vi "MESLog_Detail_Result.vi"(0 "DetailResultID":string, 1 "ItemResultID":string, 2 "Barcode":string, 3 "LoopID":string, 4 "BeginDate":string, 5 "DiffTime":string, 6 "EndDate":string, 7 "Description":string, 8 "DetailResult":string, 10 "CreateDate":string) -> (16 "Detail_Result":string)   [LabVIEW 2014]
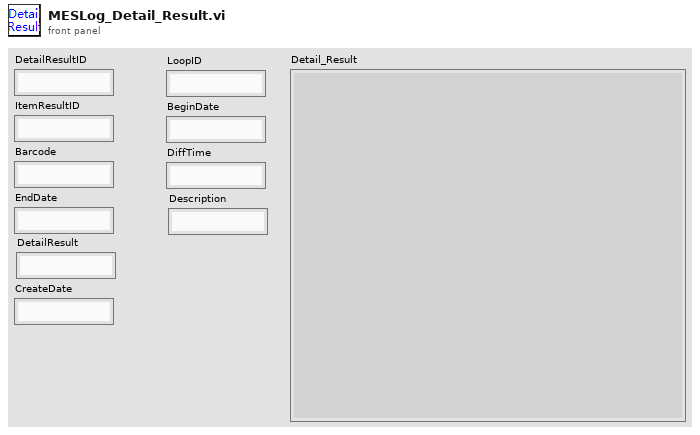
[diagram p1: front panel]
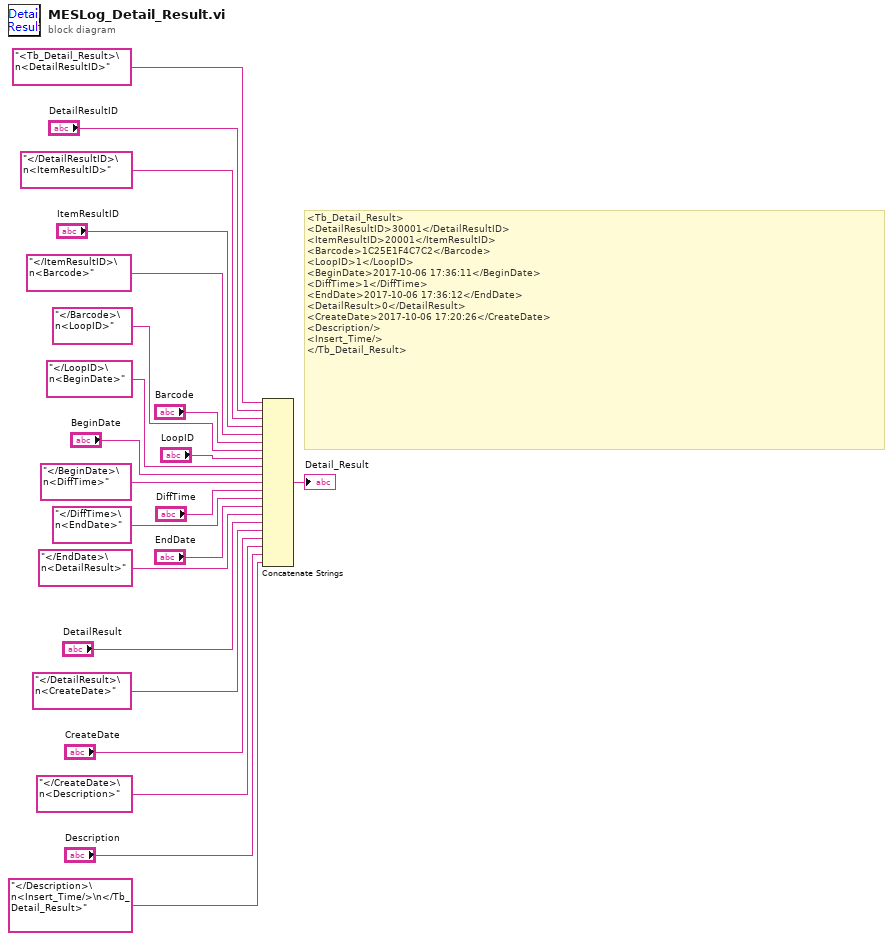
[diagram p0: block diagram]
diagram:
  # "<Tb_Detail_Result>\n<DetailResultID>30001</DetailResultID>\n<ItemResultID>20001</ItemResultID>\n<Barcode>1C25E1F4C7C2</Barcode>\n<LoopID>1</LoopID>\n<BeginDate>2017-10-06 17:36:11</BeginDate>\n<DiffTime>1</DiffTime>\n<EndDate>2017-10-06 17:36:12</EndDate>\n<DetailResult>0</DetailResult>\n<CreateDate>2017-10-06 17:20:26</CreateDate>\n<Description/>\n<Insert_Time/>\n</Tb_Detail_Result>"
  n1 = Concatenate Strings("<Tb_Detail_Result>\n<DetailResultID>" ("string"), "DetailResultID", "</DetailResultID>\n<ItemResultID>" ("string"), "ItemResultID", "</ItemResultID>\n<Barcode>" ("string"), "Barcode", "</Barcode>\n<LoopID>" ("string"), "LoopID", "</LoopID>\n<BeginDate>" ("string"), "BeginDate", "</BeginDate>\n<DiffTime>" ("string"), "DiffTime", "</DiffTime>\n<EndDate>" ("string"), "EndDate", "</EndDate>\n<DetailResult>" ("string"), "DetailResult", "</DetailResult>\n<CreateDate>" ("string"), "CreateDate", "</CreateDate>\n<Description>" ("string"), "Description", "</Description>\n<Insert_Time/>\n</Tb_Detail_Result>" ("string")) -> (→"Detail_Result":string)
